vi "transitionOn.vi"(8 "Outside Counter":i32, 9 "Full On Time":i32, 10 "Slope Start Time":i32) -> (2 "Transition Gain":dbl)   [LabVIEW 2010, in "kevLib2010.lvlib"]
uses:
  kevLib2010.lvlib
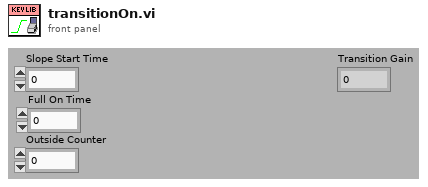
[diagram p1: front panel]
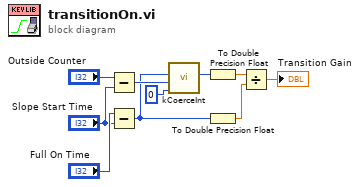
[diagram p0: block diagram]
diagram:
  n1 = Subtract(x="Outside Counter", y="Slope Start Time") -> (x-y=w6:i32)
  n2 = Subtract(x="Full On Time", y="Slope Start Time") -> (x-y=w4:i32)
  n3 = call "kCoerceInt.vi"("lower"=0, "input"=w6, "upper"=w4) -> ("output"=w5:i32)  [unwired: 7 in, 1 out]
  n4 = To Double Precision Float(number=w5) -> (double precision float=w3:dbl)
  n5 = To Double Precision Float(number=w4) -> (double precision float=w2:dbl)
  n6 = Divide(x=w3, y=w2) -> (x/y=→"Transition Gain":dbl)
